vi "Get Path Regex.vi"(8 "error in (no error)":errorcluster, 11 "CurrentStateController in":refnum<class "CurrentStateController.lvclass">) -> (0 "error out":errorcluster, 2 "Path Regex":string, 3 "CurrentStateController out":refnum<class "CurrentStateController.lvclass">)   [LabVIEW 2022 SP3, in "VideoMux.lvlib" / "CurrentStateController.lvclass"]
uses:
  CurrentStateController.lvclass
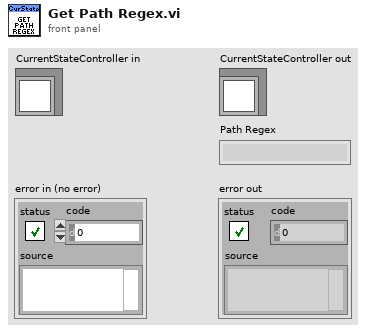
[diagram p1: front panel]
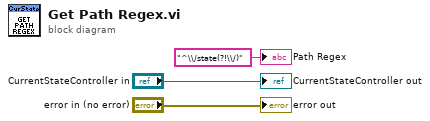
[diagram p0: block diagram]
diagram:
  "error out" <- "error in (no error)"
  "CurrentStateController out" <- "CurrentStateController in"
  "Path Regex" <- "^\\/state(?!\\/)" ("Path Regex")
